vi "Update Counter Signals.vi"(8 "error in (no error)":errorcluster, 9 "Overrides":dbl[](array[numeric]), 10 "Protections":T1, 11 "Frame Settings in":T2 {"Protection Configurations"."CRC Channels"."Data Type" items=["Signed", "Unsigned", "IEEE Float"]}) -> (0 "error out":errorcluster, 1 "Overrides out":dbl[](array[numeric]), 2 "Protections out":T1, 3 "Frame Settings out":T2 {"Protection Configurations"."CRC Channels"."Data Type" items=["Signed", "Unsigned", "IEEE Float"]})   [LabVIEW 2019, in "Protection and Counter Support Engine.lvlib"]
uses:
  Protection and Counter Support Engine.lvlib
  Types/RT Frame Settings.ctl
  Shared/Types/Exported Frame Type.ctl
  Types/RT Protection Configuration.ctl
  Shared/Types/Protection Type.ctl
  Shared/Types/XNET Signal Configuration.ctl
  Shared/Types/Exported Counter Settings.ctl
  Shared/Types/Exported Event Trigger Type.ctl
  <vilib>/NI/NIVS Inline Async API/_Data Access Engine/Data Access Engine/Types/Write.DVR.ctl
  <vilib>/NI/NIVS Inline Async API/_Data Access Engine/Access Type Classes/Write/Write.lvclass
  <vilib>/NI/NIVS Inline Async API/_Data Access Engine/Access Type Classes/Write/Write.lvclass/Write.ctl
  <vilib>/NI/NIVS Inline Async API/_Data Access Engine/Data Access Engine/Methods/Data.Processes.Execute.vi
  <vilib>/NI/NIVS Inline Async API/_Data Access Engine/Data Access Engine/Methods/Write.Data.Buffer.vi
  <vilib>/NI/NIVS Inline Async API/_Data Access Engine/Access Type Classes/Write/Write.Buffer.vi
  Shared/Protection and Counter Support Shared.lvlib
  <vilib>/NI/NIVS Inline Async API/_Data Access Engine/Data Access Engine/Data Access Engine.lvclass
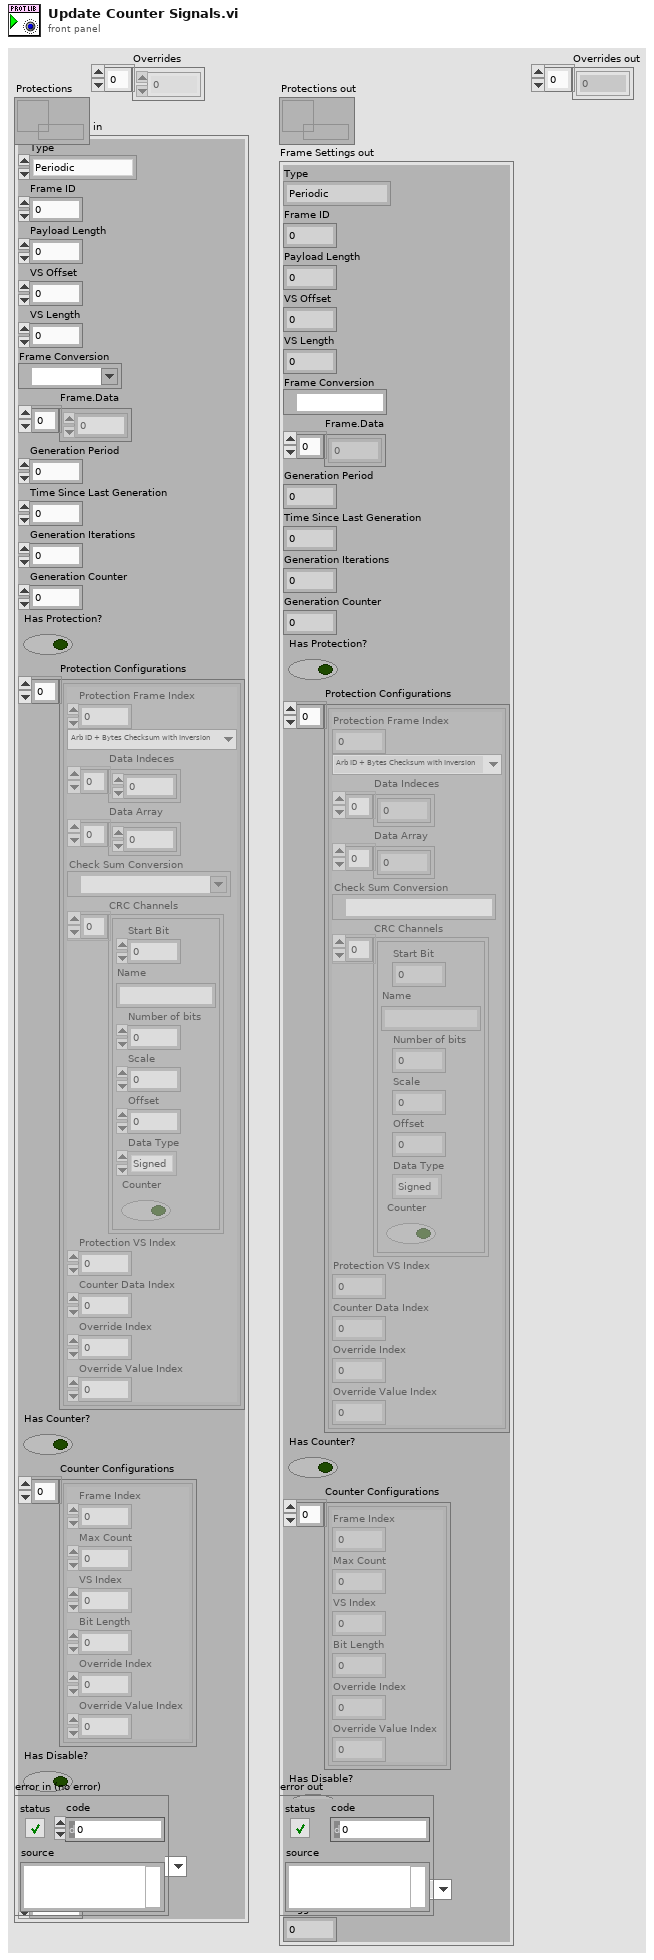
[diagram p1: front panel]
types:
  T1 = typedef "Data Access Engine.lvlib/Data Access Engine.lvclass/Write.DVR.ctl" = refnum<data-value>
  T2 = typedef "Protection and Counter Support Engine.lvlib/RT Frame Settings.ctl" = cluster{"Type":T3, "Frame ID":u32, "Payload Length":u32, "VS Offset":i32, "VS Length":i32, "Frame Conversion":refnum<k21>, "Frame.Data":dbl[], "Generation Period":u32, "Time Since Last Generation":u32, "Generation Iterations":u32, "Generation Counter":u32, "Has Protection?":bool, "Protection Configurations":T4[], "Has Counter?":bool, "Counter Configurations":T7[], "Has Disable?":bool, "Disable VS Index":i32, "Transmit Trigger":T8, "Trigger VS Index":i32}
  T3 = typedef "Protection and Counter Support Shared.lvlib/Exported Frame Type.ctl" = enum16{"Periodic", "Event", "Periodic/Event"}
  T4 = typedef "Protection and Counter Support Engine.lvlib/RT Protection Configuration.ctl" = cluster{"Protection Frame Index":i32, "Protection Type":T5, "Data Indeces":i32[], "Data Array":dbl[], "Check Sum Conversion":refnum<k21>, "CRC Channels":T6[], "Protection VS Index":i32, "Counter Data Index":i32, "Override Index":i32, "Override Value Index":i32}
  T5 = typedef "Protection and Counter Support Shared.lvlib/Protection Type.ctl" = enum16{"Arb ID + Bytes Checksum with Inversion", "Arb ID + Bytes CRC with Inversion", "Reversed Raw Signal Checksum with Inversion", "Concatenated Two's Compliment"}
  T6 = typedef "Protection and Counter Support Shared.lvlib/XNET Signal Configuration.ctl" = cluster{"Start Bit":i32, "Name":string, "Number of bits":i32, "Scale":dbl, "Offset":dbl, "Data Type":u32, "Counter":bool}
  T7 = typedef "Protection and Counter Support Shared.lvlib/Exported Counter Settings.ctl" = cluster{"Frame Index":i32, "Max Count":dbl, "VS Index":i32, "Bit Length":i64, "Override Index":i32, "Override Value Index":i32}
  T8 = typedef "Protection and Counter Support Shared.lvlib/Exported Event Trigger Type.ctl" = enum16{"Channel value change", "Trigger channel (not zero)", "Channel value change or trigger channel (not zero)", "Trigger channel (any value change)", "Channel value change or trigger channel (any value change)"}
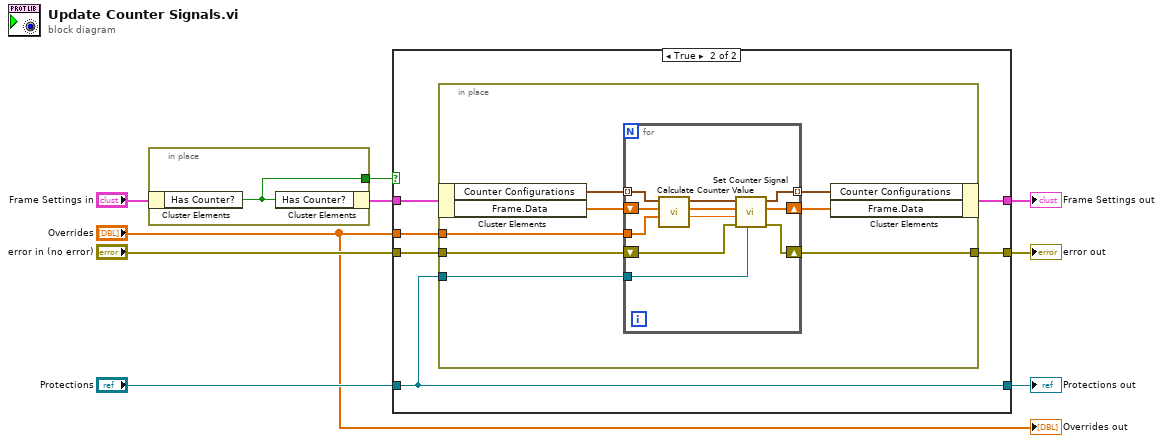
[diagram p0: block diagram]
diagram:
  n1 = in-place {
    in-place-border: [w10] -> w2
    n2 = in-place-cluster #1("Frame Settings in") -> ("Has Counter?"=w10:bool)
    n3 = in-place-cluster #1("Has Counter?"=w10) -> (w3:T2)
  }
  n4 = case shown="True" w2 {
    tunnel: "error in (no error)" -> [w13 w19]
    tunnel: [w13 w18] -> w6
    tunnel: "Protections" -> [w12 w17]
    tunnel: [w12 w17] -> w8
    tunnel: w3 -> [w11 w16]
    tunnel: [w11 w15] -> w9
    tunnel: "Overrides" -> [_ w14]
    frame False {
    }
    frame True {
      n5 = in-place {
        in-place-border: w19 -> [w27]
        in-place-border: [w26] -> w18
        in-place-border: w17 -> [w25]
        in-place-border: w14 -> [w20]
        n6 = in-place-cluster #2(w16) -> ("Counter Configurations"=w24:T7[], "Frame.Data"=w21:dbl[])
        n7 = for {
          shift-right: [w34] -> w22
          shift-left: w21 -> [w30]
          tunnel: w24 -> [w31] mode=indexing
          shift-right: [w37] -> w26
          shift-left: w27 -> [w38]
          tunnel: w25 -> [w33]
          tunnel: [w35] -> w23 mode=indexing
          tunnel: w20 -> [w28]
          n8 = call "Calculate Counter Value.vi"("Overrides"=w28, "Frame.Data in"=w30, "Counter Configuration in"=w31) -> ("Counter Value"=w36:dbl, "Frame.Data out"=w29:dbl[], "Counter Configuration out"=w32:T7)  [unwired: 6 in]
          n9 = call "Set Counter Signal.vi"("Protections"=w33, "error in (no error)"=w38, "Counter Value"=w36, "Frame.Data in"=w29, "Counter Configuration in"=w32) -> ("error out"=w37:errorcluster, "Frame.Data out"=w34:dbl[], "Counter Configuration out"=w35:T7)  [unwired: 4 in]
        }
        n10 = in-place-cluster #2("Counter Configurations"=w23, "Frame.Data"=w22) -> (w15:T2)
      }
    }
  }
  "Frame Settings out" <- w9
  "Protections out" <- w8
  "error out" <- w6
  "Overrides out" <- "Overrides"
